vi "Set_Roadblock.vi"(0 "Set_Obstacles(X, Y)":dbl[][](array[numeric])) -> (1 "Posi_Roadblock_Bound":dbl[][](array[numeric]), 2 "Posi_Roadblock":dbl[][](array[numeric]))   [LabVIEW 2020]
panel:
  # "X_Bottom, Y_Left\n\nX_Upper, Y_Right"
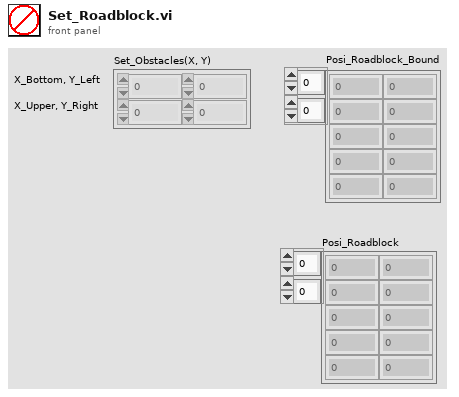
[diagram p1: front panel]
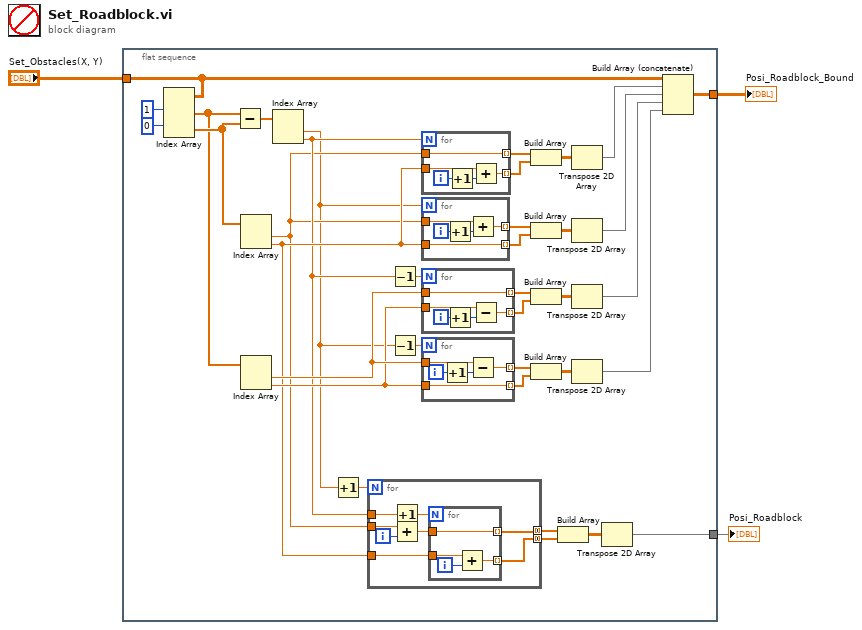
[diagram p0: block diagram]
diagram:
  n1 = flat-sequence {
    tunnel: "Set_Obstacles(X, Y)" -> [w21]
    tunnel: [w13] -> w2
    tunnel: [w5] -> w1
    frame #0 {
      n2 = Index Array(array=w21, index (row) #1=1 ("index (row)"), index (row) #2=0 ("index (row)")) -> (element #1=w24:dbl[], element #2=w37:dbl[])  [unwired: 2 in]
      n3 = Subtract(x=w24, y=w37) -> (x-y=w16:dbl[])
      n4 = Index Array(array=w37) -> (element #1=w10:dbl, element #2=w12:dbl)  [unwired: 2 in]
      n5 = Index Array(array=w24) -> (element #1=w18:dbl, element #2=w17:dbl)  [unwired: 2 in]
      n6 = Index Array(array=w16) -> (element #1=w9:dbl, element #2=w11:dbl)  [unwired: 2 in]
      n7 = Increment(x=w9) -> (x+1=w4:dbl)
      n8 = for {
        N: w4 -> [_]
        tunnel: w12 -> [w46]
        tunnel: w11 -> [w47]
        tunnel: w10 -> [w45]
        tunnel: [w41] -> w8 mode=concatenating
        tunnel: [w42] -> w7 mode=concatenating
        i -> [w43]
        n9 = Increment(x=w47) -> (x+1=w40:dbl)
        n10 = Add(x=w45, y=w43) -> (x+y=w44:dbl)
        n11 = for {
          N: w40 -> [_]
          tunnel: [w51] -> w42 mode=indexing
          tunnel: w46 -> [w50]
          tunnel: w44 -> [w49]
          tunnel: [w49] -> w41 mode=indexing
          i -> [w48]
          n12 = Add(x=w50, y=w48) -> (x+y=w51:dbl)
        }
      }
      n13 = Decrement(x=w11) -> (x-1=w15:dbl)
      n14 = Decrement(x=w9) -> (x-1=w14:dbl)
      n15 = for {
        N: w11 -> [_]
        tunnel: [w70] -> w19 mode=indexing
        tunnel: w12 -> [w69]
        tunnel: [w68] -> w20 mode=indexing
        tunnel: w10 -> [w68]
        i -> [w71]
        n16 = Increment(x=w71) -> (x+1=w67:i32)
        n17 = Add(x=w69, y=w67) -> (x+y=w70:dbl)
      }
      n18 = for {
        N: w9 -> [_]
        tunnel: [w65] -> w36 mode=indexing
        tunnel: w10 -> [w64]
        tunnel: [w63] -> w35 mode=indexing
        tunnel: w12 -> [w63]
        i -> [w66]
        n19 = Increment(x=w66) -> (x+1=w62:i32)
        n20 = Add(x=w64, y=w62) -> (x+y=w65:dbl)
      }
      n21 = for {
        N: w15 -> [_]
        tunnel: [w61] -> w26 mode=indexing
        tunnel: w17 -> [w60]
        tunnel: [w59] -> w25 mode=indexing
        tunnel: w18 -> [w59]
        i -> [w58]
        n22 = Increment(x=w58) -> (x+1=w57:i32)
        n23 = Subtract(x=w60, y=w57) -> (x-y=w61:dbl)
      }
      n24 = for {
        N: w14 -> [_]
        tunnel: [w56] -> w27 mode=indexing
        tunnel: w18 -> [w55]
        tunnel: [w54] -> w28 mode=indexing
        tunnel: w17 -> [w54]
        i -> [w53]
        n25 = Increment(x=w53) -> (x+1=w52:i32)
        n26 = Subtract(x=w55, y=w52) -> (x-y=w56:dbl)
      }
      n27 = Build Array(w20, w19) -> (w34:dbl[][])
      n28 = Build Array(w36, w35) -> (w33:dbl[][])
      n29 = Build Array(w25, w26) -> (w29:dbl[][])
      n30 = Build Array(w27, w28) -> (w30:dbl[][])
      n31 = Build Array(w8, w7) -> (w6:dbl[][])
      n32 = Transpose 2D Array(2D array=w34) -> (transposed array=w32:dbl[][])
      n33 = Transpose 2D Array(2D array=w33) -> (transposed array=w31:dbl[][])
      n34 = Transpose 2D Array(2D array=w29) -> (transposed array=w23:dbl[][])
      n35 = Transpose 2D Array(2D array=w30) -> (transposed array=w22:dbl[][])
      n36 = Transpose 2D Array(2D array=w6) -> (transposed array=w5:dbl[][])
      n37 = Build Array (concatenate)(w21, w32, w31, w23, w22) -> (w13:dbl[][])
    }
  }
  "Posi_Roadblock_Bound" <- w2
  "Posi_Roadblock" <- w1
